vi "Build Sensor Set.vi"(10 "Distance":i32, 11 "Point":T1) -> (3 "Sensor Set Out":set{T1}(c389))   [LabVIEW 2020]
uses:
  Cluster _Point.ctl
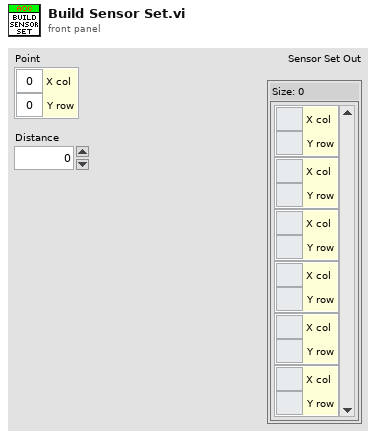
[diagram p1: front panel]
types:
  T1 = typedef "Cluster _Point.ctl" = cluster{"X col":i32, "Y row":i32}
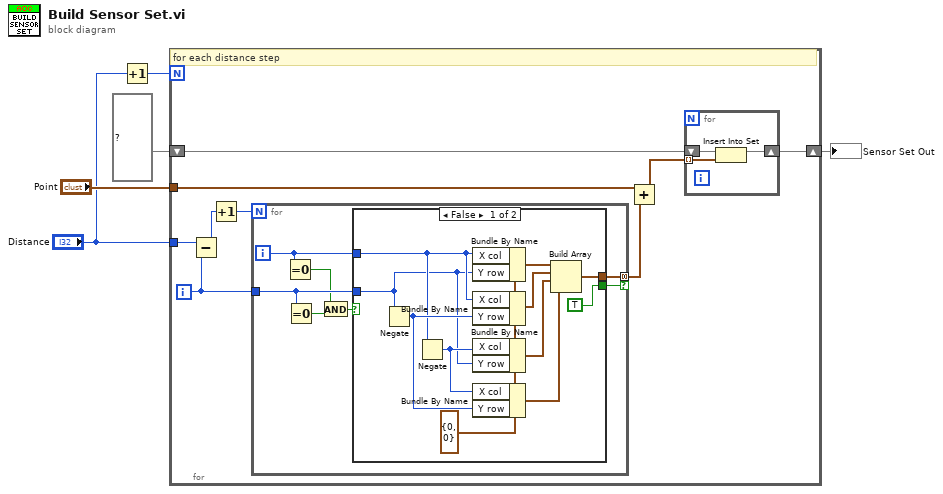
[diagram p0: block diagram]
diagram:
  n1 = Increment(x="Distance") -> (x+1=w3:i32)
  n2 = for {
    N: w3 -> [_]
    tunnel: "Point" -> [w11]
    tunnel: "Distance" -> [w14]
    shift-right: [w12] -> w2
    shift-left: set{T1} {} ("Set") -> [w13]
    i -> [w9]
    # "for each distance step"
    n3 = Subtract(x=w14, y=w9) -> (x-y=w8:i32)
    n4 = Increment(x=w8) -> (x+1=w7:i32)
    n5 = for {
      N: w7 -> [_]
      tunnel: [w24] -> w10 mode=concatenating if=w18
      tunnel: w9 -> [w22]
      i -> [w23]
      n6 = Equal To 0?(x=w23) -> (x = 0?=w20:bool)
      n7 = Equal To 0?(x=w22) -> (x = 0?=w21:bool)
      n8 = And(x=w20, y=w21) -> (x .and. y?=w19:bool)
      n9 = case shown="False" w19 {
        tunnel: [w35 _] -> w24
        tunnel: w23 -> [w27 _]
        tunnel: w22 -> [w26 _]
        tunnel: [TRUE _] -> w18
        frame False {
          w34 = T1 {"X col"=0, "Y row"=0} ("Point")
          n10 = Negate(x=w26) -> (-x=w33:i32)
          n11 = Negate(x=w27) -> (-x=w32:i32)
          n12 = Bundle By Name(cluster=w34, "X col"=w27, "Y row"=w26) -> (w31:T1)
          n13 = Bundle By Name(cluster=w34, "X col"=w27, "Y row"=w33) -> (w30:T1)
          n14 = Bundle By Name(cluster=w34, "X col"=w32, "Y row"=w26) -> (w29:T1)
          n15 = Bundle By Name(cluster=w34, "X col"=w32, "Y row"=w33) -> (w28:T1)
          n16 = Build Array(w31, w30, w29, w28) -> (w35:T1[])
        }
        frame True {
        }
      }
    }
    n17 = Add(x=w11, y=w10) -> (x+y=w6:T1[])
    n18 = for {
      shift-right: [w16] -> w12
      shift-left: w13 -> [w17]
      tunnel: w6 -> [w15] mode=indexing
      n19 = Insert Into Set(10:w15, 11:w17) -> (3:w16:set{T1})  [unwired: 1 out]
    }
  }
  "Sensor Set Out" <- w2
